vi "Main On Load Action VI.vi"(8 "error in (no error)":errorcluster, 11 "Device Item Ref in":T1 format="%.0x") -> (0 "error out":errorcluster, 3 "Device Item Ref out":T1 format="%.0x")   [LabVIEW 2016, in "Ballard Arinc-429 System Explorer.lvlib"]
uses:
  Ballard Arinc-429 System Explorer.lvlib
  <vilib>/NI Veristand/Custom Device API/Custom Device Item Ref.ctl
  <vilib>/NI VeriStand/Custom Device API/Custom Device API.lvlib
  <vilib>/NI Veristand/Custom Device API/Path Type.ctl
  <vilib>/NI Veristand/Custom Device API/Path Specification.ctl
  <vilib>/NI Veristand/Custom Device API/Custom Device Supported Target.ctl
  <vilib>/NI Veristand/Custom Device API/Custom Device Path Data.ctl
  <vilib>/NI Veristand/Custom Device API/Custom Device Execution Mode.ctl
  NationalInstruments.VeriStand.SystemDefinitionAPI
  Shared/Controls and Global/Global.vi
  Shared/Ballard Arinc-429 Shared.lvlib
  <vilib>/NI Veristand/Custom Device API/Get Item Property (Variant).vi
  <vilib>/NI Veristand/Custom Device API/Set Item Property (Variant).vi
  Shared/Controls and Global/Specify module by.ctl
  <vilib>/NI Veristand/Custom Device API/Set Item Property (U16).vi
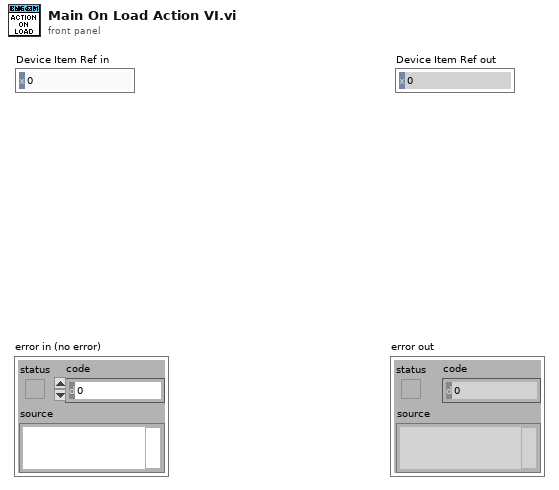
[diagram p1: front panel]
types:
  T1 = typedef "Custom Device API.lvlib/Custom Device Item Ref.ctl" = u64
  T2 = typedef "Custom Device API.lvlib/Path Specification.ctl" = cluster{"Path":path, "Type":T3}
  T3 = typedef "Custom Device API.lvlib/Path Type.ctl" = enum16{"Absolute", "To Base", "To Common Data Dir", "To Application Data Dir"}
  T4 = typedef "Custom Device API.lvlib/Custom Device Execution Mode.ctl" = enum16{"Asynchronous", "Inline HW Interface", "Inline Model Interface", "Inline Timing and Sync", "Asynchronous Timing and Sync"}
  T5 = typedef "Custom Device API.lvlib/Custom Device Supported Target.ctl" = enum16{"All", "PharLap", "VxWorks", "Windows", "Linux_32_ARM", "Linux_x64", "PharLap & Windows", "PharLap & VxWorks", "VxWorks & Windows"}
  T6 = typedef "Custom Device API.lvlib/Custom Device Path Data.ctl" = cluster{"SupportedTarget":T5, "Source":T2, "RT Destination":path}
  T7 = typedef "Ballard Arinc-429 Shared.lvlib/Specify module by.ctl" = enum16{"Index", "SlotID", "Serial number"}
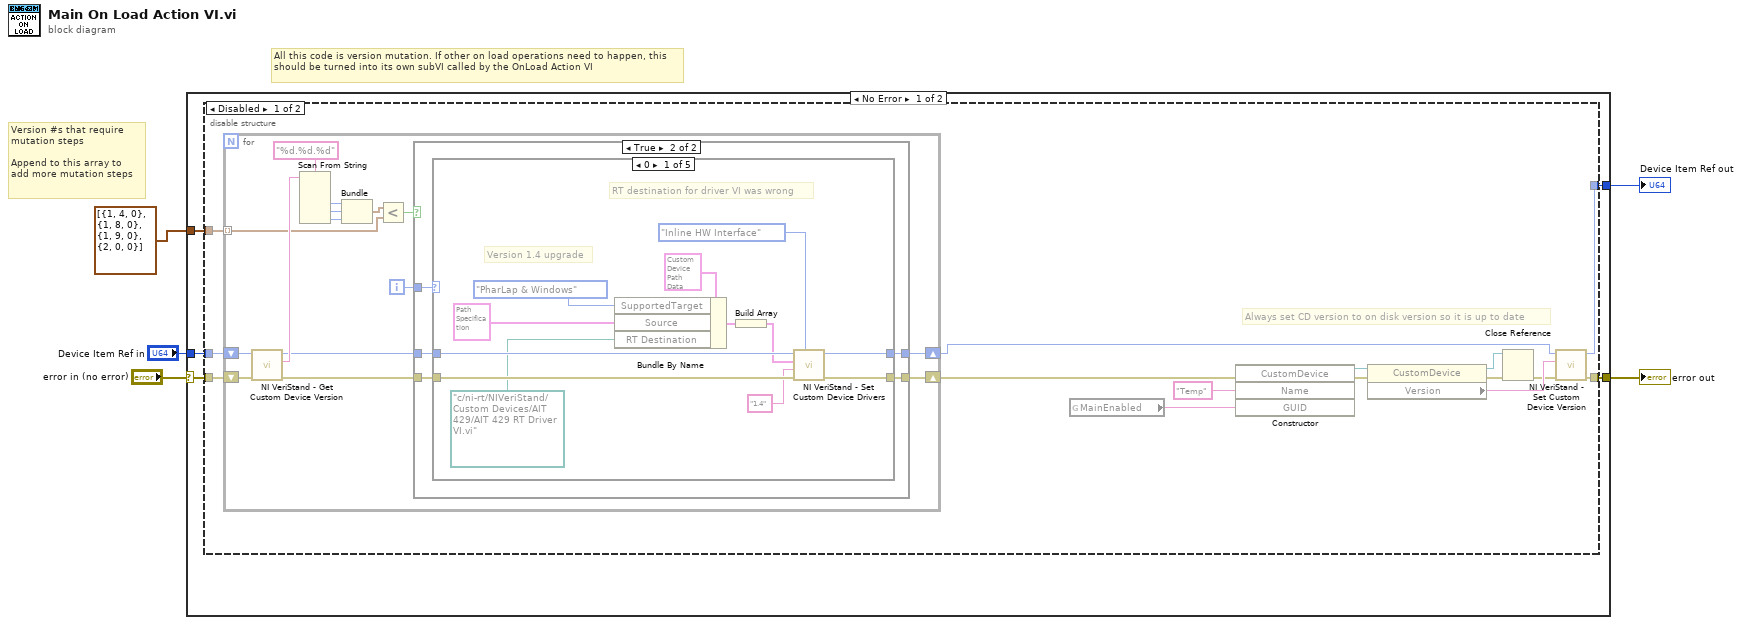
[diagram p0: block diagram]
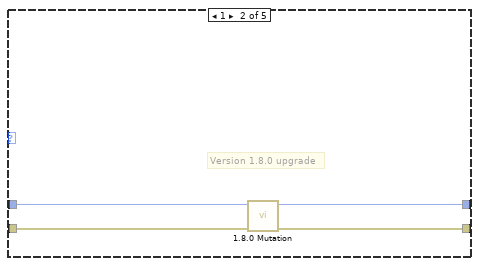
[diagram p3: hidden frame]
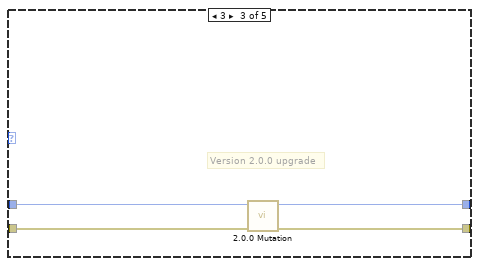
[diagram p4: hidden frame]
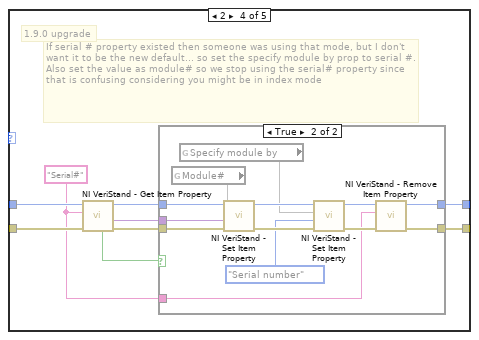
[diagram p5: hidden frame]
diagram:
  # "All this code is version mutation. If other on load operations need to happen, this should be turned into its own subVI called by the OnLoad Action VI"
  # "Version #s that require\nmutation steps\n\nAppend to this array to\nadd more mutation steps"
  n1 = case shown="No Error" "error in (no error)" {
    selector: "error in (no error)" -> [w9 w96]
    tunnel: [w7 w96] -> w4
    tunnel: "Device Item Ref in" -> [w8 w95]
    tunnel: [w6 w95] -> w2
    tunnel: cluster{i32, i32, i32}[] [{1, 4, 0}, {1, 8, 0}, {1, 9, 0}, {2, 0, 0}] -> [w10 _]
    frame No Error {
      n2 = disable-structure shown="Disabled" {
        disable-tunnel: w10 -> [w25 _]
        disable-tunnel: w9 -> [w24 w94]
        disable-tunnel: w8 -> [w23 _]
        disable-tunnel: [w13 w94] -> w7
        disable-tunnel: [w12 _] -> w6
        frame Disabled {
          # "Always set CD version to on disk version so it is up to date"
          n3 = for {
            tunnel: w25 -> [w27] mode=indexing
            shift-right: [w31] -> w21
            shift-left: w24 -> [w36]
            shift-right: [w29] -> w22
            shift-left: w23 -> [w35]
            i -> [w28]
            n4 = call <vilib>:"NI VeriStand - Get Custom Device Version.vi"("error in (no error)"=w36, "Device Ref in"=w35) -> ("error out"=w32:errorcluster, "Value"=w34:string, "Device Ref out"=w30:T1)  [unwired: 7 in]
            n5 = Scan From String(format string="%d.%d.%d", input string=w34) -> (output 1=w38:i32, output 2=w39:i32, output 3=w26:i32)  [unwired: 5 in, 3 out]
            n6 = Bundle(w38, w39, w26) -> (w40:cluster{i32, i32, i32})  [unwired: 1 in]
            n7 = Less?(x=w40, y=w27) -> (x < y?=w33:bool)
            n8 = case shown="True" w33 {
              tunnel: w32 -> [w42 w47]
              tunnel: [w42 w46] -> w31
              tunnel: w30 -> [w41 w43]
              tunnel: [w41 w44] -> w29
              tunnel: w28 -> [_ w45]
              frame False {
              }
              frame True {
                n9 = case shown="0" w45 {
                  tunnel: w47 -> [w57 w63 w67 w76 w93]
                  tunnel: [w49 w61 w65 w70 w93] -> w46
                  tunnel: [w59 w60 w64 w69 w92] -> w44
                  tunnel: w43 -> [w56 w62 w66 w75 w92]
                  frame 0 {
                    # "RT destination for driver VI was wrong"
                    # "Version 1.4 upgrade"
                    n10 = Bundle By Name(cluster=T6 {"SupportedTarget"=enum."All", "Source"={"Path"=path "", "Type"=enum."Absolute"}, "RT Destination"=path ""} ("Driver VI Path"), "SupportedTarget"=Custom_Device_Supported_Target."PharLap & Windows", "Source"=T2 {"Path"=path "Custom Devices/AIT 429/AIT 429 RT Driver VI.vi", "Type"=enum."To Common Data Dir"}, "RT Destination"=path "c:/ni-rt/NIVeriStand/Custom Devices/AIT 429/AIT 429 RT Driver VI.vi") -> (w54:T6)
                    n11 = Build Array(w54) -> (w53:T6[])
                    n12 = call <vilib>:"NI VeriStand - Set Custom Device Drivers.vi"("Execution mode"=Custom_Device_Execution_Mode."Inline HW Interface", "error in (no error)"=w57, "Version"="1.4" ("format string"), "Driver VI"=w53, "Device Ref in"=w56) -> ("error out"=w49:errorcluster, "Device Ref out"=w59:T1)  [unwired: 5 in]
                  }
                  frame 1 {
                    # "Version 1.8.0 upgrade"
                    n13 = call "1.8.0 Mutation.vi"("error in"=w63, "Device Ref in"=w62) -> ("error out"=w61:errorcluster, "Device Ref out"=w60:T1)  [unwired: 8 in]
                  }
                  frame 3 {
                    # "Version 2.0.0 upgrade"
                    n14 = call "2.0.0 Mutation.vi"("error in"=w67, "Device Ref in"=w66) -> ("error out"=w65:errorcluster, "Device Ref out"=w64:T1)  [unwired: 8 in]
                  }
                  frame 2 {
                    w68 = "Serial#" ("x")
                    # "If serial # property existed then someone was using that mode, but I don't want it to be the new default... so set the specify module by prop to serial #. Also set the value as module# so we stop using the serial# property since that is confusing considering you might be in index mode"
                    # "1.9.0 upgrade"
                    n15 = call-poly <vilib>:"NI VeriStand - Get Item Property.vi"("error in (no error)"=w76, "Property Name"=w68, "Item Ref in"=w75) -> ("error out"=w73:errorcluster, "Value"=w71:variant, "Item Ref out"=w72:T1, "Found?"=w74:bool)  [unwired: 5 in]
                    n16 = case shown="True" w74 {
                      tunnel: w73 -> [w77 w91]
                      tunnel: w72 -> [w78 w90]
                      tunnel: w71 -> [_ w88]
                      tunnel: [w77 w82] -> w70
                      tunnel: [w78 w80] -> w69
                      tunnel: w68 -> [_ w79]
                      frame False {
                      }
                      frame True {
                        n17 = global read "Global.vi" "Module#"() -> (w89)
                        n18 = global read "Global.vi" "Specify module by"() -> (w85)
                        n19 = call-poly <vilib>:"NI VeriStand - Set Item Property.vi"("error in (no error)"=w91, "Value"=w88, "Property Name"=w89, "Item Ref in"=w90) -> ("error out"=w86:errorcluster, "Item Ref out"=w87:T1)  [unwired: 5 in, 1 out]
                        n20 = call-poly <vilib>:"NI VeriStand - Set Item Property.vi"("error in (no error)"=w86, "Value"=Specify_module_by."Serial number" ("Specify module by"), "Property Name"=w85, "Item Ref in"=w87) -> ("error out"=w83:errorcluster, "Item Ref out"=w81:T1)  [unwired: 5 in, 1 out]
                        n21 = call <vilib>:"NI VeriStand - Remove Item Property.vi"("error in (no error)"=w83, "Property Name"=w79, "Item Ref in"=w81) -> ("error out"=w82:errorcluster, "Item Ref out"=w80:T1)  [unwired: 6 in, 1 out]
                      }
                    }
                  }
                  frame Default {
                  }
                }
              }
            }
          }
          n22 = global read "Global.vi" "MainEnabled"() -> (w11:string)
          n23 = constructor class="CustomDevice"(error in=w21, "Name"="Temp", "GUID"=w11) -> (reference out=w19:refnum<k24>, error out=w18:errorcluster)  [unwired: 2 in, 3 out]
          n24 = property class="CustomDevice"(reference=w19, error in=w18) -> (reference out=w16:refnum<k24>, error out=w17:errorcluster, "Version"=w15:string)
          n25 = Close Reference(reference=w16, error in (no error)=w17) -> (error out=w14:errorcluster)
          n26 = call <vilib>:"NI VeriStand - Set Custom Device Version.vi"("error in (no error)"=w14, "Value"=w15, "Device Ref in"=w22) -> ("error out"=w13:errorcluster, "Device Ref out"=w12:T1)  [unwired: 7 in]
        }
        frame Enabled {
        }
      }
    }
    frame Error {
    }
  }
  "error out" <- w4
  "Device Item Ref out" <- w2
